vi "test encoding.vi"() -> ()   [LabVIEW 2020]
uses:
  FaceRecognitionDotNet/FaceRecognition Class/ctl/LocationModel.ctl
  FaceRecognitionDotNet/FaceRecognition Class/FaceRecognition.lvclass
panel:
  in  "mode path":path=path "F:/MY FILE/FaceRecognitionDotNet 1.2.3.10/FaceRecognitionDotNet/models"
  out "FaceDistance 2":dbl
  out "FaceDistance":dbl
  in  "face 2":path
  in  "face 1":path
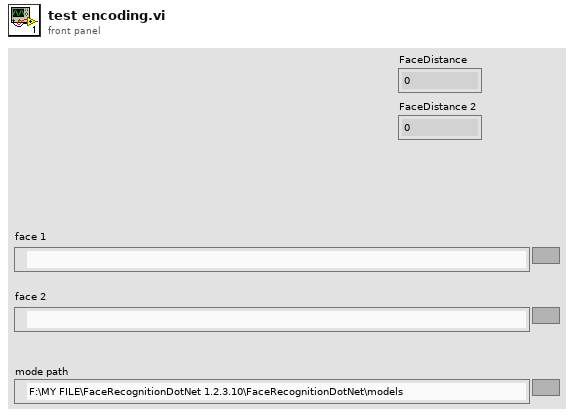
[diagram p1: front panel]
types:
  T1 = enum16{"open", "replace", "create", "open or create", "replace or create", "replace or create with confirmation"}
  T2 = typedef "FaceRecognitionDotNet.lvlib/FaceRecognition.lvclass/LocationModel.ctl" = i32
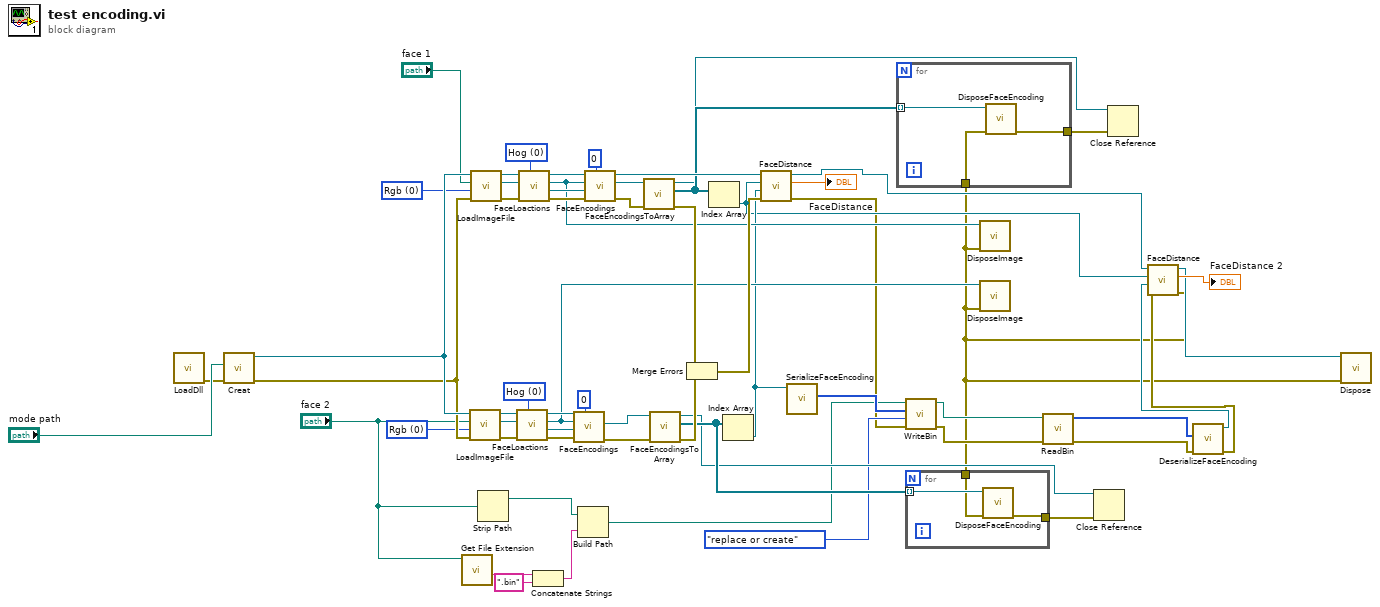
[diagram p0: block diagram]
diagram:
  w46 = T2 0 items=["Hog", "Cnn"] ("model")
  w47 = 0 items=["Rgb", "Greyscale"] ("mode")
  w53 = T2 0 items=["Hog", "Cnn"] ("model")
  w57 = 0 items=["Rgb", "Greyscale"] ("mode")
  n1 = call "LoadDll.vi"() -> ("error out"=w60:errorcluster)  [unwired: 11 in]
  n2 = call "Creat.vi"("error in (no error)"=w60, "mode path"="mode path") -> ("error out"=w58:errorcluster, "FaceRecognition out"=w59:refnum<class "FaceRecognition.lvclass">)  [unwired: 8 in]
  n3 = call <vilib>:"Get File Extension.vi"("file"="face 2") -> ("filename without extension"=w7:string)  [unwired: 6 in, 4 out]
  n4 = call "LoadImageFile.vi"("error in (no error)"=w58, "mode"=w47, "FilePath"="face 2", "FaceRecognition in"=w59) -> ("error out"=w45:errorcluster, "LoadImageFile"=w44:refnum<k24>, "FaceRecognition out"=w43:refnum<class "FaceRecognition.lvclass">)  [unwired: 5 in]
  n5 = call "LoadImageFile.vi"("error in (no error)"=w58, "mode"=w57, "FilePath"="face 1", "FaceRecognition in"=w59) -> ("error out"=w54:errorcluster, "LoadImageFile"=w50:refnum<k24>, "FaceRecognition out"=w55:refnum<class "FaceRecognition.lvclass">)  [unwired: 5 in]
  n6 = Strip Path(path="face 2") -> (stripped path=w4:path)  [unwired: 1 out]
  n7 = call "FaceLoactions.vi"("model"=w46, "error in (no error)"=w45, "image"=w44, "FaceRecognition in"=w43) -> ("error out"=w41:errorcluster, "FaceLocations"=w40:refnum<k24>, "image out"=w29:refnum<k24>, "FaceRecognition out"=w39:refnum<class "FaceRecognition.lvclass">)  [unwired: 4 in]
  n8 = call "FaceLoactions.vi"("model"=w53, "error in (no error)"=w54, "image"=w50, "FaceRecognition in"=w55) -> ("error out"=w49:errorcluster, "FaceLocations"=w51:refnum<k24>, "image out"=w30:refnum<k24>, "FaceRecognition out"=w48:refnum<class "FaceRecognition.lvclass">)  [unwired: 4 in]
  n9 = Concatenate Strings(w7, ".bin" ("string")) -> (w3:string)
  n10 = call "FaceEncodings.vi"("numJitters"=0, "error in (no error)"=w41, "knownFaceLocation"=w40, "image"=w29, "FaceRecognition in"=w39) -> ("error out"=w36:errorcluster, "FaceEncodings"=w1:refnum<k24>)  [unwired: 4 in, 1 out]
  n11 = Build Path(base path=w4, name or relative path=w3) -> (appended path=w2:path)
  n12 = call "FaceEncodings.vi"("numJitters"=0, "error in (no error)"=w49, "knownFaceLocation"=w51, "image"=w30, "FaceRecognition in"=w48) -> ("error out"=w37:errorcluster, "FaceEncodings"=w38:refnum<k24>, "FaceRecognition out"=w32:refnum<class "FaceRecognition.lvclass">)  [unwired: 4 in]
  n13 = call "FaceEncodingsToArray.vi"("error in (no error)"=w37, "FaceEncodings in"=w38) -> ("error out"=w35:errorcluster, "FaceEncodingArray"=w28:refnum<k24>[], "FaceEncodings out"=w23:refnum<k24>)  [unwired: 7 in]
  n14 = call "FaceEncodingsToArray.vi"("error in (no error)"=w36, "FaceEncodings in"=w1) -> ("error out"=w34:errorcluster, "FaceEncodingArray"=w27:refnum<k24>[], "FaceEncodings out"=w26:refnum<k24>)  [unwired: 7 in]
  n15 = Merge Errors(w35, w34) -> (w33:errorcluster)
  n16 = Index Array(array=w28) -> (element=w16:refnum<k24>)  [unwired: 1 in]
  n17 = Index Array(array=w27) -> (element=w22:refnum<k24>)  [unwired: 1 in]
  n18 = call "FaceDistance.vi"("error in (no error)"=w33, "faceToCompare"=w22, "FaceEncoding"=w16, "FaceRecognition in"=w32) -> ("error out"=w8:errorcluster, "FaceDistance"=→"FaceDistance":dbl, "FaceRecognition out"=w18:refnum<class "FaceRecognition.lvclass">)  [unwired: 5 in]
  n19 = call "SerializeFaceEncoding.vi"("FaceEncoding in"=w22) -> ("BinaryEncoding"=w20:u8[])  [unwired: 8 in, 2 out]
  n20 = call "WriteBin.vi"("error in (no error)"=w8, "operation (0:open)"=T1."replace or create", "BinaryEncoding"=w20, "appended path"=w2) -> ("error out"=w14:errorcluster, "path"=w15:path)  [unwired: 6 in]
  n21 = call "ReadBin.vi"("error in (no error)"=w14, "FaceEncoding file"=w15) -> ("error out"=w12:errorcluster, "Array"=w13:u8[])  [unwired: 8 in]
  n22 = call "DeserializeFaceEncoding.vi"("error in (no error)"=w12, "BinaryEncoding"=w13) -> ("error out"=w10:errorcluster, "FaceEncoding"=w11:refnum<k24>)  [unwired: 8 in]
  n23 = call "FaceDistance.vi"("error in (no error)"=w10, "faceToCompare"=w11, "FaceEncoding"=w16, "FaceRecognition in"=w18) -> ("error out"=w9:errorcluster, "FaceDistance"=→"FaceDistance 2":dbl, "FaceRecognition out"=w17:refnum<class "FaceRecognition.lvclass">)  [unwired: 5 in]
  n24 = for {
    tunnel: w28 -> [w64] mode=indexing
    tunnel: w9 -> [w63]
    tunnel: [w62] -> w24
    n25 = call "DisposeFaceEncoding.vi"("error in (no error)"=w63, "FaceEncoding in"=w64) -> ("error out"=w62:errorcluster)  [unwired: 9 in]
  }
  n26 = for {
    tunnel: w27 -> [w67] mode=indexing
    tunnel: w9 -> [w66]
    tunnel: [w65] -> w25
    n27 = call "DisposeFaceEncoding.vi"("error in (no error)"=w66, "FaceEncoding in"=w67) -> ("error out"=w65:errorcluster)  [unwired: 9 in]
  }
  n28 = call "DisposeImage.vi"("error in (no error)"=w9, "Image in"=w30) -> ()  [unwired: 9 in, 1 out]
  n29 = call "DisposeImage.vi"("error in (no error)"=w9, "Image in"=w29) -> ()  [unwired: 9 in, 1 out]
  n30 = Close Reference(reference=w26, error in (no error)=w25) -> ()  [unwired: 1 out]
  n31 = Close Reference(reference=w23, error in (no error)=w24) -> ()  [unwired: 1 out]
  n32 = call "Dispose.vi"("error in (no error)"=w9, "FaceRecognition in"=w17) -> ()  [unwired: 8 in, 2 out]
